vi "Network Connection Handler.vi"(10 "FPGA Ref":T1, 11 "Network Info":T2 {"Last Comm Time" format="%<%H:%M:%S%3u\n%Y/%m/%d>T"; "Remote Port" format="%.0x"}) -> (0 "error out":errorcluster, 3 "connection ID out":refnum<k5>)   [LabVIEW 2023]
doc: "Author: Scott Hannahs <sth@magnet.fsu.edu>\nCopyright 2018 Florida State University, All rights reserved."
uses:
  RT Controls/Network Info.ctl
  RT Controls/RT System Auth Level.ctl
  RT Controls/FPGA SCH Digitizer Ref.ctl
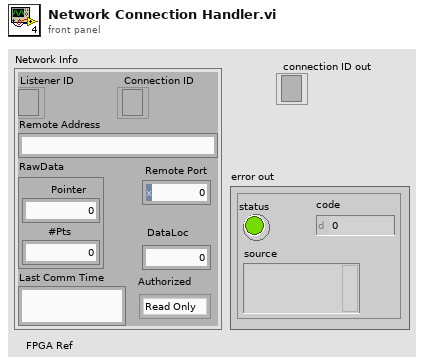
[diagram p1: front panel]
types:
  T1 = typedef "FPGA SCH Digitizer Ref.ctl" = refnum<k20>
  T2 = typedef "Network Info.ctl" = cluster{"Listener ID":refnum<k5>, "Connection ID":refnum<k5>, "Remote Address":string, "Remote Port":u16, "DataLoc":u32, "RawData":cluster{"#Pts":u32, "Pointer":u32}, "Last Comm Time":timestamp, "Authorized":T3}
  T3 = typedef "RT System Auth Level.ctl" = enum16{"Read Only", "Operator", "Admin"}
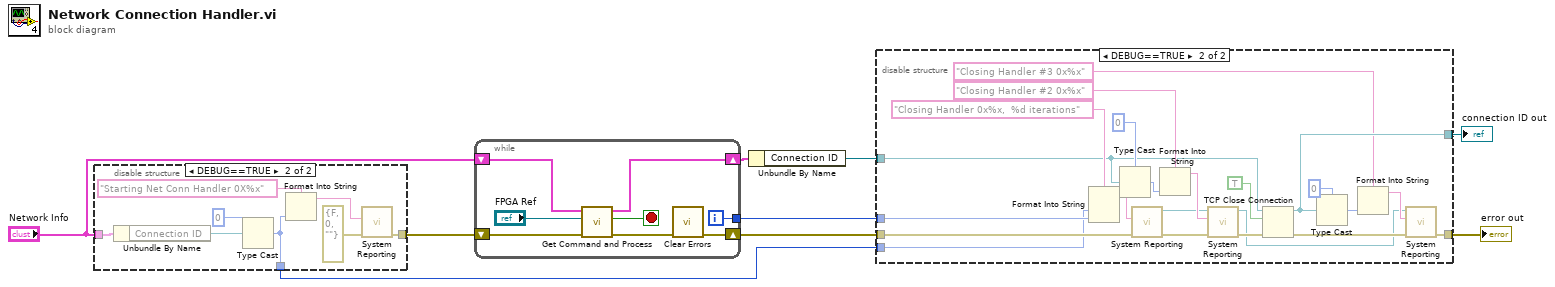
[diagram p0: block diagram]
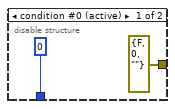
[diagram p2: hidden frame]
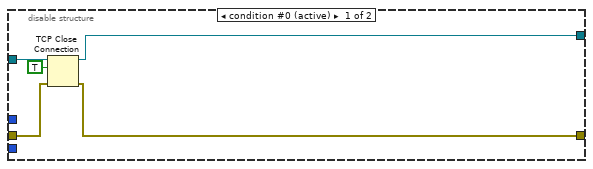
[diagram p3: hidden frame]
diagram:
  n1 = disable-structure shown="DEBUG==TRUE" {
    disable-tunnel: [errorcluster {"status"=FALSE, "code"=0, "source"=""} ("Error Out") w18] -> w8
    disable-tunnel: [u32 0 w14] -> w5
    disable-tunnel: "Network Info" -> [_ w13]
    frame condition #0 (active) {
    }
    frame condition #1 {
      n2 = Unbundle By Name(w13) -> ("Connection ID"=w12:refnum<k5>)
      n3 = Type Cast(type=u32 0, x=w12) -> (*(type *) &x=w14:u32)
      n4 = Format Into String(format string="Starting Net Conn Handler 0X%x" ("String"), w14) -> (resulting string=w17:string)  [unwired: 2 in, 1 out]
      n5 = call "System Reporting.vi"("Error In"=errorcluster {"status"=FALSE, "code"=0, "source"=""} ("error out"), "String"=w17) -> ("Error Out"=w18:errorcluster)  [unwired: 8 in, 1 out]
    }
  }
  n6 = while {
    shift-right: [w24] -> w9
    shift-left: "Network Info" -> [w25]
    shift-right: [w21] -> w7
    shift-left: w8 -> [w27]
    tunnel: [w20] -> w6
    i -> [w20]
    stop <- w23 stop-if-true
    n7 = call "Get Command and Process.vi"("Error In"=w27, "FPGA Ref"="FPGA Ref", "Network Info"=w25) -> ("Error Out"=w26:errorcluster, "Connection Dormant"=w23:bool, "Network Info out"=w24:T2)  [unwired: 6 in]
    n8 = call <vilib>:"Clear Errors.vi"("error in (no error)"=w26) -> ("error out"=w21:errorcluster)  [unwired: 5 in, 1 out]
  }
  n9 = Unbundle By Name(w9) -> ("Connection ID"=w4:refnum<k5>)
  n10 = disable-structure shown="DEBUG==TRUE" {
    disable-tunnel: w7 -> [w31 w54]
    disable-tunnel: w6 -> [_ w51]
    disable-tunnel: w5 -> [_ w50]
    disable-tunnel: w4 -> [w32 w45]
    disable-tunnel: [w29 w37] -> w3
    disable-tunnel: [w30 w35] -> w2
    frame condition #0 (active) {
      n11 = TCP Close Connection(connection ID=w32, abort (F)=TRUE, error in (no error)=w31) -> (connection ID out=w29:refnum<k5>, error out=w30:errorcluster)
    }
    frame condition #1 {
      n12 = Format Into String(format string="Closing Handler 0x%x,  %d iterations", w50, w51) -> (resulting string=w52:string)  [unwired: 2 in, 1 out]
      n13 = Type Cast(type=u32 0, x=w45) -> (*(type *) &x=w44:u32)
      n14 = call "System Reporting.vi"("Error In"=w54, "String"=w52) -> ("Error Out"=w49:errorcluster, "Byte Stream File out"=w42:refnum<file>)  [unwired: 8 in]
      n15 = Format Into String(format string="Closing Handler #2 0x%x", w44) -> (resulting string=w43:string)  [unwired: 2 in, 1 out]
      n16 = call "System Reporting.vi"("Error In"=w49, "String"=w43, "Byte Stream File in"=w42) -> ("Error Out"=w48:errorcluster, "Byte Stream File out"=w36:refnum<file>)  [unwired: 7 in]
      n17 = TCP Close Connection(connection ID=w45, abort (F)=TRUE, error in (no error)=w48) -> (connection ID out=w37:refnum<k5>, error out=w38:errorcluster)
      n18 = Type Cast(type=u32 0, x=w37) -> (*(type *) &x=w40:u32)
      n19 = Format Into String(format string="Closing Handler #3 0x%x", w40) -> (resulting string=w41:string)  [unwired: 2 in, 1 out]
      n20 = call "System Reporting.vi"("Error In"=w38, "String"=w41, "Byte Stream File in"=w36) -> ("Error Out"=w35:errorcluster)  [unwired: 7 in, 1 out]
    }
  }
  "connection ID out" <- w3
  "error out" <- w2
